vi "Scan_Dialog.vi"(0 "Acquisition Unit in (0)":i32, 1 "Acquire Definition":T9={"Acquire Mode"=enum."stop", "Acquisition mode"=enum."Sampled", "Acquirer"=enum."Cleverscope", "Transfer Chans"=enum."Chan A+B", "A max scale"=5.0, "A min scale"=-5.0, "B max scale"=5.0, "B min scale"=-5.0, "A Probe"=enum."x1", "B Probe"=enum."x1", "A Coupling"=enum."DC", "B Coupling"=enum."DC", "A Bandwidth"=1, "B Bandwidth"=1, "Trigger Source"=enum."Chan A", "Trigger Amplitude"=0.0, "A Trigger Amplitude"=0.0, "B Trigger Amplitude"=0.0, "Trigger Filter"=enum."None", "Trig Slope"=FALSE, "Trigger Holdoff"=0.0, "Dig Pattern Rqd"=FALSE, "Dig Pattern"=0, "Ext Trig Threshold"=0.0, "Dig Input Threshold"=0.0, "Start Time"=-0.003, "Stop Time"=0.003, "Pre Trig Time"=0.003, "Port"=enum."Port 1", "Num divisions"=6, "Num seq frames"=1, "Num Buffers"=2, "Sig Gen Freq"=1000.0, "Sig Gen Amp"=1.0, "Sig Gen Offset"=0.0, "Sig Gen Waveform"=enum."sine", "Sig Gen Sweep"=enum."Log", "Sig Gen Func"=enum."Standard", "Sig Gen Freq 2"=1000.0, "Sig Gen Phase"=180.0, "Trig 2 Function"=enum."None", "Min Trigger Period"=1e-08, "Max trigger Period"=0.0001, "Trigger count"=1, "Trig 2 Slope"=FALSE, "Trig 2 Source Chan"=enum."Chan A", "Trig 2 Level"=0.0, "Dig Pattern 2 Rqd"=FALSE, "Dig Pattern 2"=0, "Trigger 2 Source"=enum."Trigger 1 inverted", "Waveform Averages"=0, "Value changed"=0, "Freq Span"=0.0, "Freq Res"=0.0, "Duration"=0.0, "Resolution"=0.0, "Link Port"=enum."Debug", "Ext Sample Clock"=FALSE, "F Spare 2"=FALSE, "F Spare 3"=FALSE, "F Spare 4"=FALSE, "Sampler Resolution"=enum."10 bit", "Intf Source"=enum."USB", "Update Rate"=enum."20 Frame/sec", "Transfer Size"=enum."Normal", "Sig Gen Freq Step"=0.0, "TCP Adr"=0, "TCP port"=0, "CAU Ser Num Hi"=0, "CAU Ser Num Lo"=0, "Function Number"=0.0, "Function Parameter"=0.0, "Function Result"=0.0, "Link Start"=0, "Link Timebase"=0, "Link Timer"=0, "Link Setup"=0, "Spare 1"=0.0, "Spare 2"=0.0, "Spare 3"=0.0, "Spare 4"=0.0} {"Function Result" format="%#.6p"; "Function Parameter" format="%#.6p"; "Function Number" format="%#.6p"; "TCP Adr" format="%08x"; "Sig Gen Freq Step" format="%.2f"; "Sig Gen Phase" format="%.2f"; "Sig Gen Freq 2" format="%.2f"; "Resolution" format="%#.6p"; "Duration" format="%#.6p"; "Freq Res" format="%#.6p"; "Freq Span" format="%#.6p"; "Dig Pattern 2" format="%.0x"; "Trig 2 Level" step=0.001 format="%#.6p"; "Trigger count" step=1; "Max trigger Period" min=1e-08 max=42.9 step=0.01 format="%#.6p"; "Min Trigger Period" min=1e-08 max=42.9 step=0.01 format="%#_6p"; "Sig Gen Offset" format="%.2f"; "Sig Gen Amp" format="%.2f"; "Sig Gen Freq" format="%.2f"; "B Trigger Amplitude" format="%.1p"; "A Trigger Amplitude" format="%.1p"; "B Bandwidth" format="%x"; "A Bandwidth" format="%x"; "B min scale" format="%.2p"; "B max scale" format="%.2p"; "A min scale" format="%.2p"; "A max scale" format="%.2p"; "Trigger Holdoff" format="%.1p"; "Dig Input Threshold" format="%.2f"; "Ext Trig Threshold" format="%.2f"; "Dig Pattern" format="%.0x"; "Pre Trig Time" format="%.3p"; "Start Time" format="%.2p"; "Trigger Amplitude" format="%.1p"; "Stop Time" format="%.2p"}, 2 "Replay settings":T8={"Sampling Rate"=0.0, "Samples in replay"=0, "Replay Start Time"=1000.0, "Replay Stop Time"=0.003} {"Sampling Rate" format="%.3p"; "Samples in replay" format="%.3p"; "Replay Stop Time" format="%.3p"}, 5 "File Paths":T1, 9 "Scan Options":T5, 11 "error in":errorcluster, 12 "Scan Axis Config":T6, 13 "Index Axis Config":T6) -> (15 "error out":errorcluster)   [LabVIEW 2009]
uses:
  libraries/Cscope control driver.llb/Acquire Event type.ctl
  libraries/Cscope control driver.llb/Acquire capture type.ctl
  libraries/Cscope control driver.llb/Acquire capture method.ctl
  libraries/Cscope control driver.llb/Acquirer type.ctl
  libraries/Cscope control driver.llb/Input Range.ctl
  libraries/Cscope control driver.llb/Input Coupling.ctl
  libraries/Cscope control driver.llb/Input Bandwidth.ctl
  libraries/Cscope control driver.llb/USB channel.ctl
  libraries/Cscope control driver.llb/Trigger Filter.ctl
  libraries/Cscope control driver.llb/Cscope waveform type.ctl
  libraries/Cscope control driver.llb/Trigger Period.ctl
  libraries/Cscope control driver.llb/Trigger channel.ctl
  libraries/Cscope control driver.llb/Link port types.ctl
  libraries/Cscope control driver.llb/Acquirer resolution.ctl
  libraries/Cscope control driver.llb/Intf source.ctl
  libraries/Cscope control driver.llb/Acquire transfer size.ctl
  typedefs/Cscope/ReplaySettings.ctl
  typedefs/ScanAxisCfg.ctl
  typedefs/AxisSelect_Enum.ctl
  typedefs/SweepMode_Ring.ctl
  typedefs/ScanType.ctl
  typedefs/DwellTime.ctl
  typedefs/PathCluster.ctl
  typedefs/Ultra3000/IndexSettings_Cluster.ctl
  typedefs/Ultra3000/IndexType.ctl
  typedefs/Ultra3000/Index_Numeric.ctl
  typedefs/Ultra3000/HostControlModeRing.ctl
panel:
  in  "Channel Select":enum32{"Channel A", "Channel B", "Channel A+B"}(radio)
  out "Scan Line Progress":dbl(slide) scale=0.0..100.0 scale format="%#.0f"
  out "Total Progress":dbl(slide) scale=0.0..100.0 scale format="%#.0p"
  out "Num Points":i32
  out "dt":dbl
  out "Waveform Graph":waveform(sgl)[](graph)
  out "Status":string caption="Status \nMessage"
  in  "Stop":bool
  in  "Pause":bool
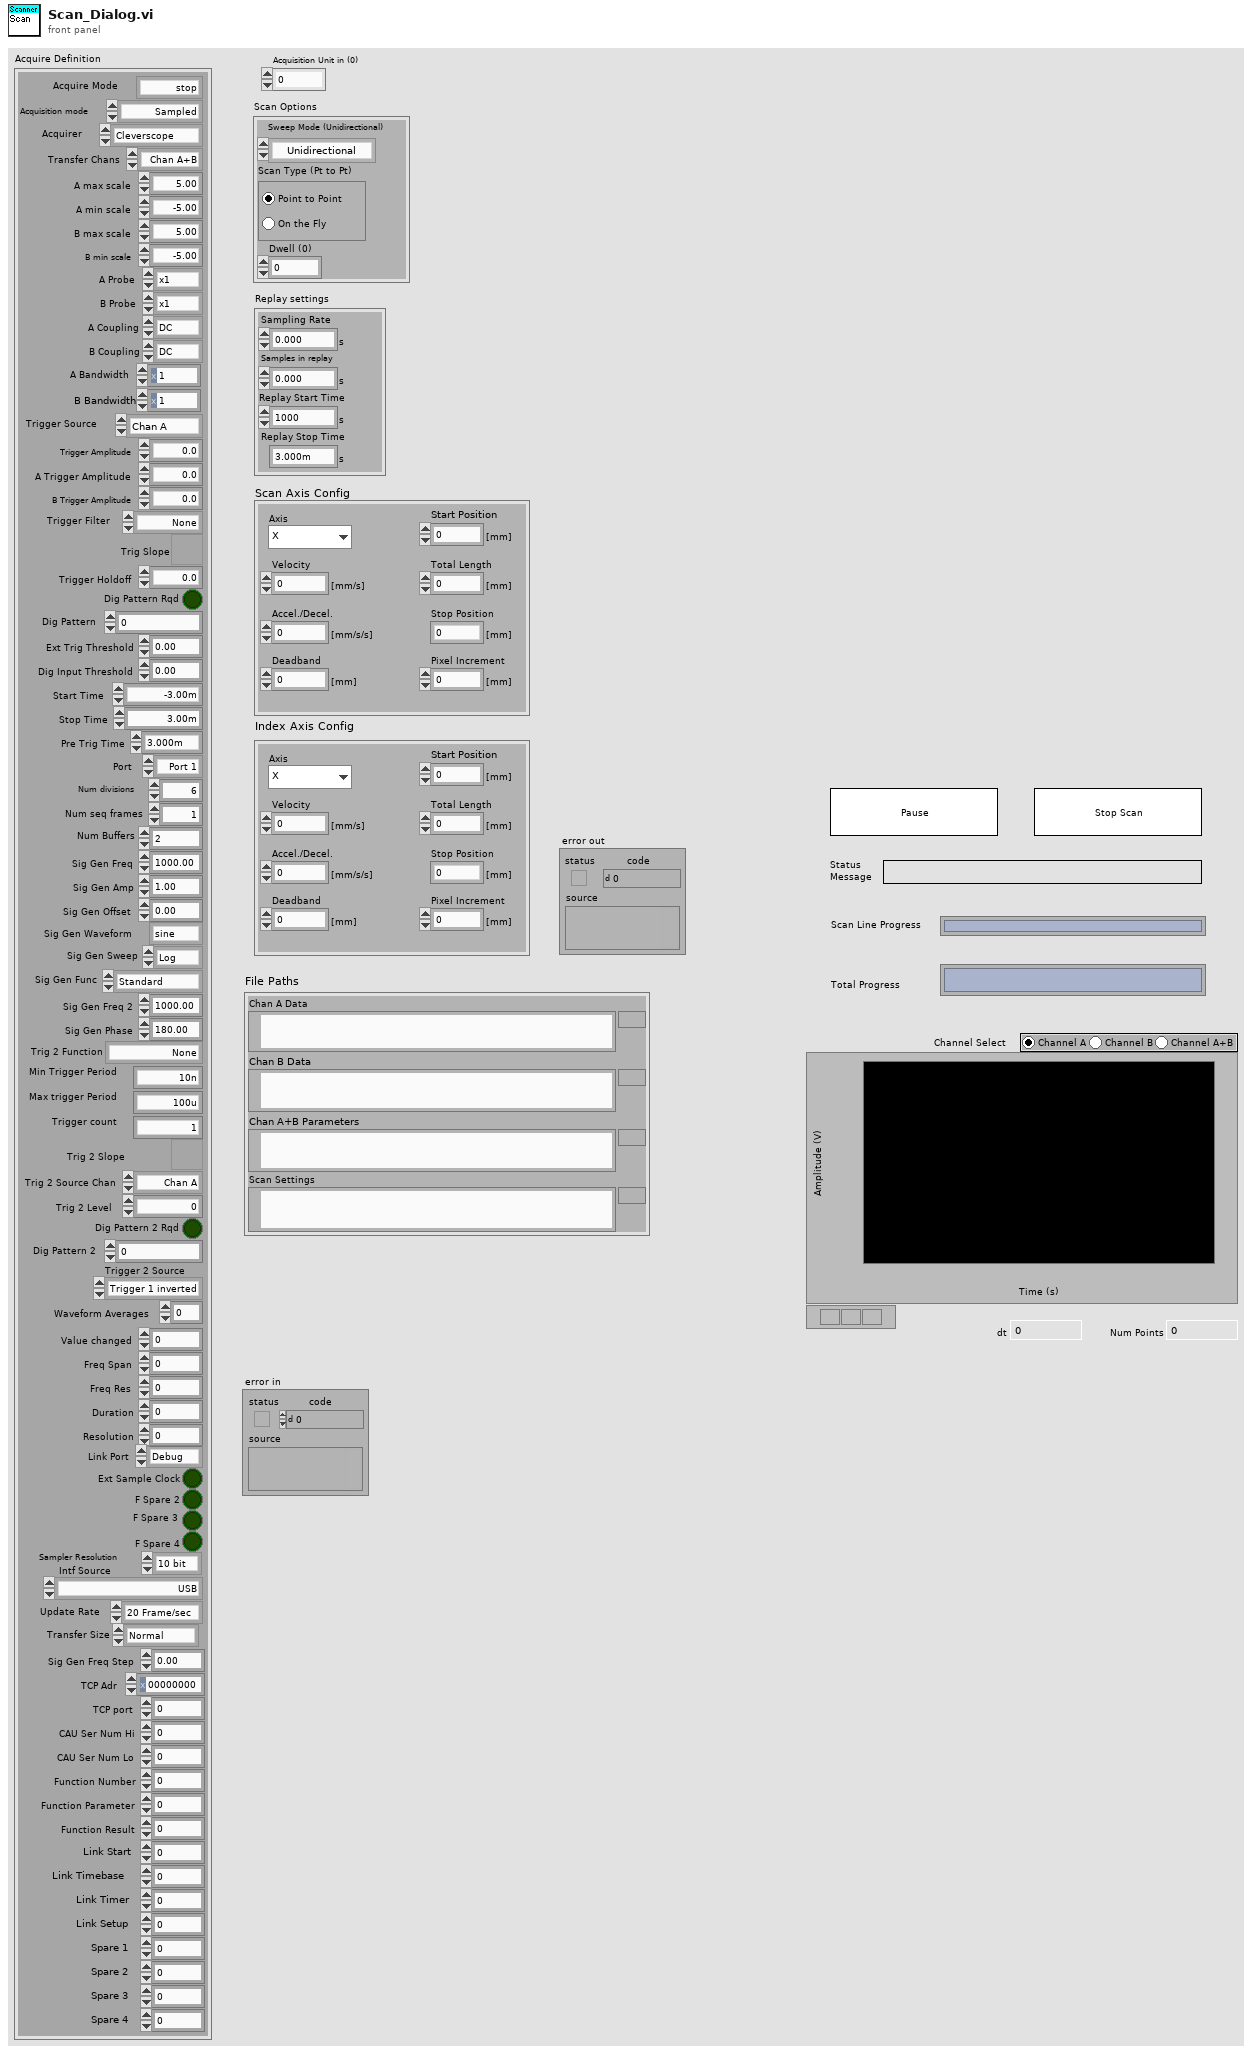
[diagram p1: front panel]
types:
  T1 = typedef "PathCluster.ctl" = cluster{"Chan A Data":path, "Chan B Data":path, "Chan A+B Parameters":path, "Scan Settings":path}
  T2 = typedef "SweepMode_Ring.ctl" = enum16{"Unidirectional", "Bidirectional"}
  T3 = typedef "ScanType.ctl" = enum32{"Point to Point", "On the Fly"}
  T4 = typedef "DwellTime.ctl" = u16
  T5 = cluster{"Sweep Mode (Unidirectional)":T2, "Scan Type (Pt to Pt)":T3, "Dwell (0)":T4}
  T6 = typedef "ScanAxisCfg.ctl" = cluster{"Axis ":T7, "Velocity":dbl, "Accel./Decel.":dbl, "Deadband":dbl, "Start Position":dbl, "Total Length":dbl, "Stop Position":dbl, "Pixel Increment":dbl}
  T7 = typedef "AxisSelect_Enum.ctl" = enum16{"X", "Y", "Z", "Axis Space"}
  T8 = typedef "ReplaySettings.ctl" = cluster{"Sampling Rate":dbl, "Samples in replay":u32, "Replay Start Time":dbl, "Replay Stop Time":dbl}
  T9 = typedef "Acquire Event type.ctl" = cluster{"Acquire Mode":T10, "Acquisition mode":T11, "Acquirer":T12, "Transfer Chans":enum16{"Chan A", "Chan B", "Chan A+B"}, "A max scale":dbl, "A min scale":dbl, "B max scale":dbl, "B min scale":dbl, "A Probe":T13, "B Probe":T13, "A Coupling":T14, "B Coupling":T14, "A Bandwidth":T15, "B Bandwidth":T15, "Trigger Source":T16, "Trigger Amplitude":dbl, "A Trigger Amplitude":dbl, "B Trigger Amplitude":dbl, "Trigger Filter":T17, "Trig Slope":bool, "Trigger Holdoff":dbl, "Dig Pattern Rqd":bool, "Dig Pattern":u32, "Ext Trig Threshold":dbl, "Dig Input Threshold":dbl, "Start Time":dbl, "Stop Time":dbl, "Pre Trig Time":dbl, "Port":enum16{"Port 1", "Port 2", "Port 3", "Port 4", "Port 5", "Port 6"}, "Num divisions":i16, "Num seq frames":i16, "Num Buffers":i32, "Sig Gen Freq":dbl, "Sig Gen Amp":dbl, "Sig Gen Offset":dbl, "Sig Gen Waveform":T18, "Sig Gen Sweep":enum16{"Linear", "Log"}, "Sig Gen Func":enum16{"Standard", "Auto advance", "Freq mod In8", "Phase mod In8"}, "Sig Gen Freq 2":dbl, "Sig Gen Phase":dbl, "Trig 2 Function":T19, "Min Trigger Period":dbl, "Max trigger Period":dbl, "Trigger count":u32, "Trig 2 Slope":bool, "Trig 2 Source Chan":T20, "Trig 2 Level":dbl, "Dig Pattern 2 Rqd":bool, "Dig Pattern 2":u32, "Trigger 2 Source":enum16{"Trigger 1 inverted", "Trig 2 Defn"}, "Waveform Averages":i32, "Value changed":i32, "Freq Span":dbl, "Freq Res":dbl, "Duration":dbl, "Resolution":dbl, "Link Port":T21, "Ext Sample Clock":bool, "F Spare 2":bool, "F Spare 3":bool, "F Spare 4":bool, "Sampler Resolution":T22, "Intf Source":T23, "Update Rate":enum16{"20 Frame/sec", "10 Frame/sec", "5 Frame/sec"}, "Transfer Size":T24, "Sig Gen Freq Step":dbl, "TCP Adr":u32, "TCP port":u32, "CAU Ser Num Hi":u32, "CAU Ser Num Lo":u32, "Function Number":dbl, "Function Parameter":dbl, "Function Result":dbl, "Link Start":u32, "Link Timebase":u32, "Link Timer":u32, "Link Setup":u32, "Spare 1":dbl, "Spare 2":dbl, "Spare 3":dbl, "Spare 4":dbl}
  T10 = typedef "Acquire capture type.ctl" = enum16{"single", "automatic", "triggered", "stop", "single stop", "replay"}
  T11 = typedef "Acquire capture method.ctl" = enum16{"Sampled", "Peak Captured", "Filtered", "Repetitive", "Waveform avg"}
  T12 = typedef "Acquirer type.ctl" = enum16{"Internal Sig Gen", "APC 901", "APC 901A", "Sound Card", "Cleverscope"}
  T13 = typedef "Input Range.ctl" = enum16{"x1", "x10", "x100", "x1K", "x20", "x50", "x200"}
  T14 = typedef "Input Coupling.ctl" = enum16{"AC", "DC"}
  T15 = typedef "Input Bandwidth.ctl" = u16
  T16 = typedef "USB channel.ctl" = enum32{"Chan A", "Chan B", "Ext Trigger", "Dig Trig", "Link Input", "chan_5", "chan_6", "chan_7", "chan_8", "chan_9", "chan_10", "chan_11", "chan_12", "chan_13", "chan_14", "chan_15"}
  T17 = typedef "Trigger Filter.ctl" = enum16{"None", "Low Pass", "Hi Pass", "Noise"}
  T18 = typedef "Cscope waveform type.ctl" = enum16{"sine", "triangle", "square", "DC", "OFF"}
  T19 = typedef "Trigger Period.ctl" = enum16{"None", "Trig 1~2 < min", "min<T1~2 < max", "Trig 1~2 > max", "Count Trig 1", "Count Trig 2"}
  T20 = typedef "Trigger channel.ctl" = enum32{"Chan A", "Chan B", "Ext Trigger", "Dig Trig", "Link Input"}
  T21 = typedef "Link port types.ctl" = enum8{"Debug", "Link Out", "Disabled", "Slave", "Master", "Uart", "SPI", "I2C", "Digital", "Sig Gen"}
  T22 = typedef "Acquirer resolution.ctl" = enum16{"10 bit", "12 Bit", "14 bit"}
  T23 = typedef "Intf source.ctl" = enum16{"USB", "Ethernet - Find by IP address", "Ethernet - Find first IP address", "Ethernet - Find by serial number"}
  T24 = typedef "Acquire transfer size.ctl" = enum16{"Normal", "100% Buffer", "50% Buffer", "10% Buffer", "5% Buffer", "2% Buffer", "Sequence"}
  T25 = typedef "Index_Numeric.ctl" = u8
  T26 = typedef "IndexSettings_Cluster.ctl" = cluster{"Type":T27, "Dwell":T4, "Velocity":dbl, "Accel/Decel":dbl}
  T27 = typedef "IndexType.ctl" = i32
  T28 = typedef "HostControlModeRing.ctl" = u16
  T29 = enum16{"big-endian, network order", "native, host order", "little-endian"}
  T30 = typedef "QSig_T0dt.ctl" = cluster{"T0":dbl, "dt":dbl, "n":i32}
  T31 = typedef "Cscope real.ctl" = sgl
  T32 = cluster{"Chan A Data":T31[], "Chan B Data":T31[]}
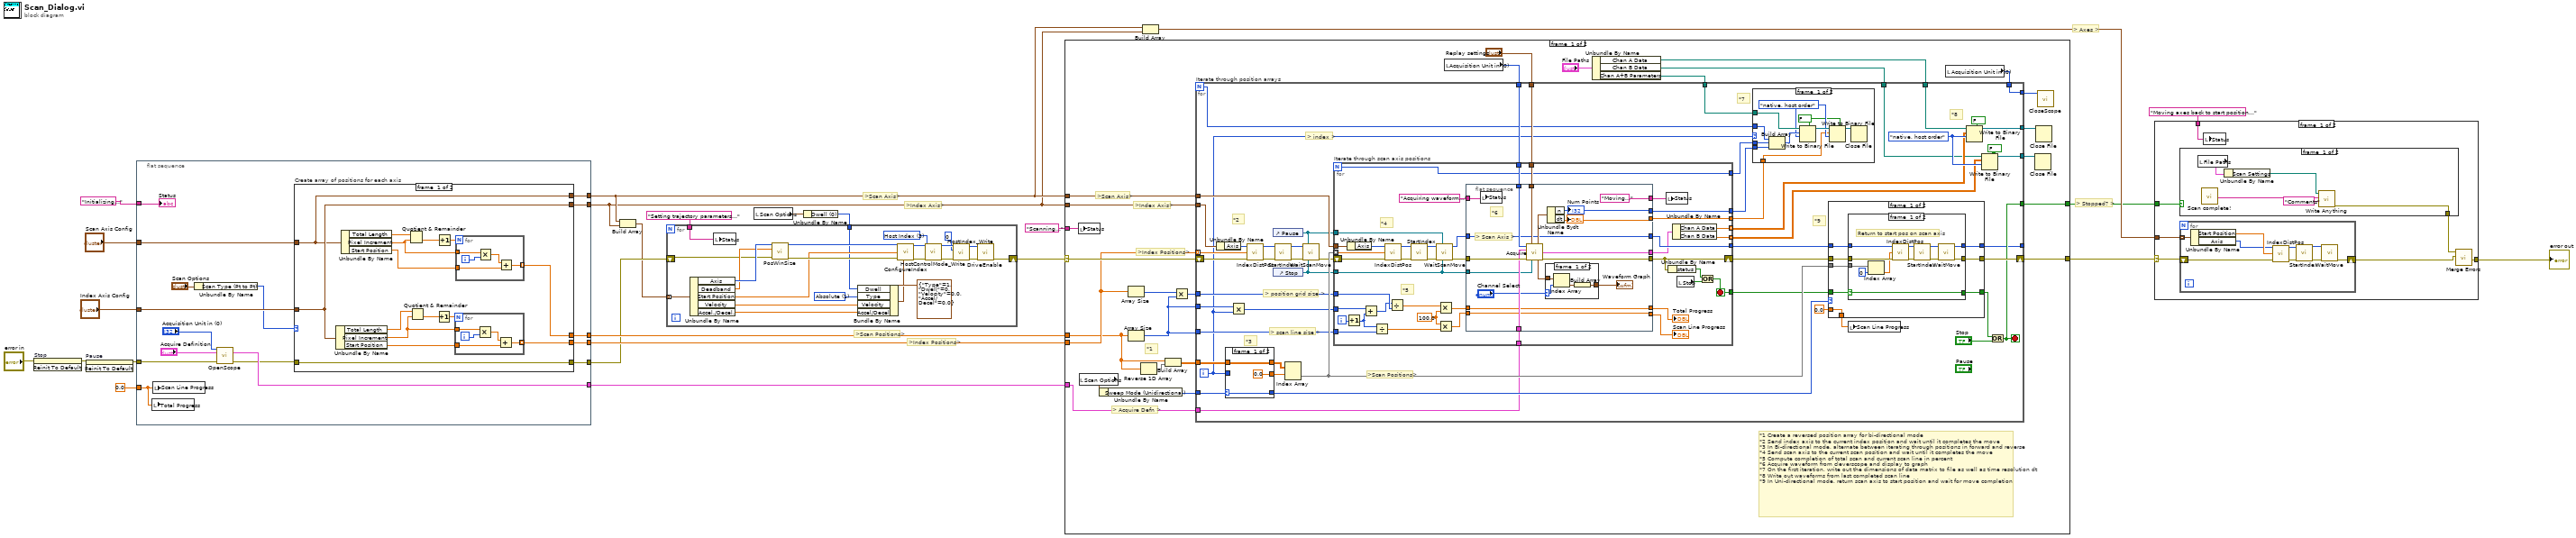
[diagram p0: block diagram]
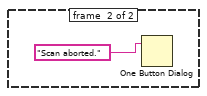
[diagram p2: hidden frame]
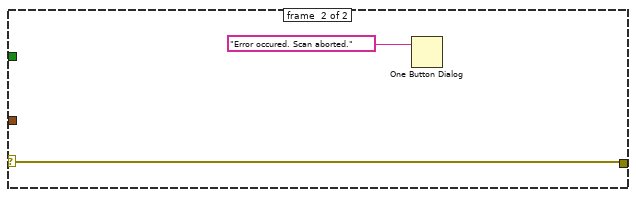
[diagram p3: hidden frame]
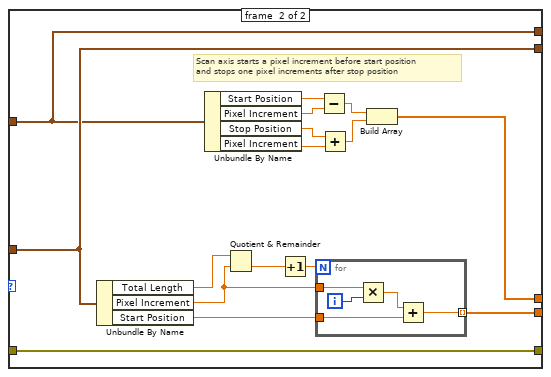
[diagram p4: hidden frame]
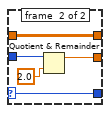
[diagram p6: hidden frame]
diagram:
  # "> Axes >"
  # "> Stopped? >"
  # ">Index Positions>"
  # ">Scan Positions>"
  # ">Index Axis>"
  # ">Scan Axis>"
  n1 = invoke on="Stop" class="Bool (strict)" method="Reinit To Default"(error in="error in") -> (error out=w5:errorcluster)  [unwired: 2 in, 2 out]
  n2 = invoke on="Pause" class="Bool (strict)" method="Reinit To Default"(error in=w5) -> (error out=w3:errorcluster)  [unwired: 2 in, 2 out]
  n3 = flat-sequence {
    tunnel: "Index Axis Config" -> [w40]
    tunnel: "Scan Axis Config" -> [w39]
    tunnel: [w38] -> w20
    tunnel: [w37] -> w19
    tunnel: [w36] -> w21
    tunnel: [w35] -> w22
    tunnel: [w32] -> w18
    tunnel: [w33] -> w6
    tunnel: "Initializing..." ("Status") -> [w31]
    tunnel: w3 -> [w29]
    tunnel: 0.0 ("Scan Line Progress") -> [w25]
    frame #0 {
      n4 = local write "Total Progress"(w25) -> ()
      n5 = local write "Scan Line Progress"(w25) -> ()
      n6 = Unbundle By Name("Scan Options") -> ("Scan Type (Pt to Pt)"=w26:T3)
      n7 = call "OpenScope.vi"("Acquisition Unit in (0)"="Acquisition Unit in (0)", "Acquire Defn In"="Acquire Definition", "error in"=w29) -> ("Acquire Defn Out"=w33:T9, "error out"=w28:errorcluster)  [unwired: 9 in, 2 out]
      n8 = case "Create array of positions for each axis" shown="\"Point to Point\", Default" w26 {
        tunnel: w40 -> [w45 w80]
        tunnel: w39 -> [w44 w79]
        tunnel: [w42 w81] -> w37
        tunnel: [w41 w66] -> w38
        tunnel: [w45 w80] -> w36
        tunnel: [w44 w79] -> w35
        tunnel: w28 -> [w43 w67]
        tunnel: [w43 w67] -> w32
        frame #0 {
          n9 = Unbundle By Name(w45) -> ("Total Length"=w49:dbl, "Pixel Increment"=w46:dbl, "Start Position"=w51:dbl)
          n10 = Unbundle By Name(w44) -> ("Total Length"=w53:dbl, "Pixel Increment"=w47:dbl, "Start Position"=w55:dbl)
          n11 = Quotient & Remainder(x=w53, y=w47) -> (floor(x/y)=w52:dbl)  [unwired: 1 out]
          n12 = Quotient & Remainder(x=w49, y=w46) -> (floor(x/y)=w48:dbl)  [unwired: 1 out]
          n13 = Increment(x=w48) -> (x+1=w50:dbl)
          n14 = Increment(x=w52) -> (x+1=w54:dbl)
          n15 = for {
            N: w50 -> [_]
            tunnel: w51 -> [w59]
            tunnel: w46 -> [w57]
            tunnel: [w56] -> w41 mode=indexing
            i -> [w60]
            n16 = Multiply(x=w57, y=w60) -> (x*y=w58:dbl)
            n17 = Add(x=w58, y=w59) -> (x+y=w56:dbl)
          }
          n18 = for {
            N: w54 -> [_]
            tunnel: w55 -> [w64]
            tunnel: w47 -> [w62]
            tunnel: [w61] -> w42 mode=indexing
            i -> [w65]
            n19 = Multiply(x=w62, y=w65) -> (x*y=w63:dbl)
            n20 = Add(x=w63, y=w64) -> (x+y=w61:dbl)
          }
        }
        frame #1 {
          # "Scan axis starts a pixel increment before start position \nand stops one pixel increments after stop position"
          n21 = Unbundle By Name(w80) -> ("Total Length"=w70:dbl, "Pixel Increment"=w69:dbl, "Start Position"=w68:dbl)
          n22 = Unbundle By Name(w79) -> ("Start Position"=w75:dbl, "Pixel Increment"=w74:dbl, "Stop Position"=w77:dbl, "Pixel Increment"=w78:dbl)
          n23 = Quotient & Remainder(x=w70, y=w69) -> (floor(x/y)=w71:dbl)  [unwired: 1 out]
          n24 = Increment(x=w71) -> (x+1=w72:dbl)
          n25 = for {
            N: w72 -> [_]
            tunnel: w68 -> [w85]
            tunnel: w69 -> [w83]
            tunnel: [w82] -> w66 mode=indexing
            i -> [w86]
            n26 = Multiply(x=w83, y=w86) -> (x*y=w84:dbl)
            n27 = Add(x=w84, y=w85) -> (x+y=w82:dbl)
          }
          n28 = Subtract(x=w75, y=w74) -> (x-y=w73:dbl)
          n29 = Add(x=w77, y=w78) -> (x+y=w76:dbl)
          n30 = Build Array(w73, w76) -> (w81:dbl[])
        }
      }
      "Status" <- w31
    }
  }
  n31 = Build Array(w22, w21) -> (w14:T6[])
  n32 = local read "Scan Options"() -> (w9:T5)
  n33 = Unbundle By Name(w9) -> ("Dwell (0)"=w8:T4)
  n34 = for {
    tunnel: w14 -> [w107] mode=indexing
    shift-right: [w91] -> w23
    shift-left: w18 -> [w90]
    tunnel: "Setting trajectory parameters..." ("Status") -> [w88]
    tunnel: w8 -> [w87]
    w92 = T28 3 items=["Normal Mode", "Setpoint velocity", "Setpoint current", "Host Index"] ("Host Control Mode (Normal)")
    w89 = T27 1 items=["Incremental", "Absolute", "Registration", "Jog"] ("Type")
    n35 = Unbundle By Name(w107) -> ("Axis"=w106:T7, "Deadband"=w104:dbl, "Start Position"=w100:dbl, "Velocity"=w101:dbl, "Accel./Decel."=w102:dbl)
    n36 = local write "Status"(w88) -> ()
    n37 = call "PosWinSize.vi"("Axis In"=w106, "Position Window Size"=w104, "error in (no error)"=w90) -> ("Axis Out"=w105:T7, "error out"=w103:errorcluster)  [unwired: 11 in]
    n38 = Bundle By Name(cluster=T26 {"Type"=1, "Dwell"=0, "Velocity"=0.0, "Accel/Decel"=0.0} ("Index Settings"), "Dwell"=w87, "Type"=w89, "Velocity"=w101, "Accel/Decel"=w102) -> (w108:T26)
    n39 = call "ConfigureIndex.vi"("Axis In"=w105, "Position"=w100, "error in (no error)"=w103, "Index Settings"=w108) -> ("Axis Out"=w98:T7, "error out"=w97:errorcluster)  [unwired: 9 in, 1 out]
    n40 = call "HostControlMode_Write.vi"("Axis In"=w98, "Host Control Mode (Normal)"=w92, "error in (no error)"=w97) -> ("Axis Out"=w99:T7, "error out"=w96:errorcluster)  [unwired: 11 in]
    n41 = call "HostIndex_Write.vi"("Axis In (Axis Space)"=w99, "Index"=T25 0, "error in (no error)"=w96) -> ("Axis Out"=w93:T7, "error out"=w94:errorcluster)  [unwired: 10 in, 1 out]
    n42 = call "DriveEnable.vi"("Axis In (Axis Space)"=w93, "error in (no error)"=w94) -> ("error out"=w91:errorcluster)  [unwired: 12 in, 1 out]
  }
  n43 = case shown="No Error" w23 {
    selector: w23 -> [w131 w296]
    tunnel: w20 -> [w124 _]
    tunnel: [w130 w296] -> w2
    tunnel: w19 -> [w123 _]
    tunnel: w21 -> [w133 _]
    tunnel: w22 -> [w132 _]
    tunnel: w6 -> [w129 _]
    tunnel: "Scanning..." ("Status") -> [w126 _]
    tunnel: [w125 _] -> w10
    frame #0 {
      # "*1"
      # "> Acquire Defn >"
      # ">Index Positions>"
      # ">Index Axis>"
      # ">Scan Axis>"
      # "*1 Create a reversed position array for bi-directional mode\n*2 Send index axis to the current index position and wait until it completes the move\n*3 In Bi-directional mode, alternate between iterating through positions in forward and reverse\n*4 Send scan axis to the current scan position and wait until it completes the move\n*5 Compute completion of total scan and current scan line in percent\n*6 Acquire waveform from cleverscope and display to graph\n*7 On the first iteration, write out the dimensions of data matrix to file as well as time resolution dt\n*8 Write out waveforms from last completed scan line\n*9 In Uni-directional mode, return scan axis to start position and wait for move completion"
      n44 = local write "Status"(w126) -> ()
      n45 = local read "Scan Options"() -> (w119:T5)
      n46 = Unbundle By Name(w119) -> ("Sweep Mode (Unidirectional)"=w118:T2)
      n47 = Array Size(array=w124) -> (size(s)=w116:i32)
      n48 = Array Size(array=w123) -> (size(s)=w115:i32)
      n49 = Reverse 1D Array(array=w123) -> (reversed array=w135:dbl[])
      n50 = Build Array(w123, w135) -> (w134:dbl[][])
      n51 = Multiply(x=w116, y=w115) -> (x*y=w122:i32)
      n52 = local read "Acquisition Unit in (0)"() -> (w127:i32)
      n53 = Unbundle By Name("File Paths") -> ("Chan A Data"=w114:path, "Chan B Data"=w113:path, "Chan A+B Parameters"=w112:path)
      n54 = local read "Acquisition Unit in (0)"() -> (w111:i32)
      n55 = for "Iterate through position arrays" {
        N -> [w147]
        tunnel: w124 -> [w186] mode=indexing
        tunnel: w133 -> [w184]
        tunnel: w132 -> [w183]
        tunnel: w134 -> [w178]
        tunnel: w118 -> [w177]
        shift-right: [w166] -> w130
        shift-left: w131 -> [w165]
        tunnel: w129 -> [w164]
        tunnel: "Replay settings" -> [w163]
        tunnel: w127 -> [w162]
        tunnel: [w159] -> w125
        tunnel: w122 -> [w158]
        tunnel: w115 -> [w157]
        tunnel: [w153] -> w121
        tunnel: [w152] -> w120
        tunnel: w112 -> [w138]
        tunnel: w115 -> [w145]
        tunnel: w114 -> [w140]
        tunnel: w113 -> [w139]
        tunnel: [w137] -> _
        tunnel: [w136] -> w110
        tunnel: w111 -> [w136]
        i -> [w144]
        stop <- w159 stop-if-true
        w156 = T29."native, host order" ("byte order (0:big-endian, network order)")
        # "> scan line size >"
        # "> position grid size >"
        # "> index >"
        # "*9"
        # "*8"
        # "*7"
        # "*3"
        # "*2"
        # ">Scan Positions>"
        n56 = Unbundle By Name(w184) -> ("Axis"=w185:T7)
        n57 = case shown="\"Bidirectional\"" w177 {
          selector: w177 -> [w197 w200]
          tunnel: w178 -> [w199 w201]
          tunnel: w144 -> [_ w203]
          tunnel: [0.0 w202] -> w176
          tunnel: [w199 w201] -> w175
          tunnel: [w197 w200] -> w173
          frame #0 {
          }
          frame #1 {
            n58 = Quotient & Remainder(x=w203, y=2.0) -> (x-y*floor(x/y)=w202:dbl)  [unwired: 1 out]
          }
        }
        n59 = Multiply(x=w145, y=w144) -> (x*y=w143:i32)
        n60 = call "IndexDistPos.vi"("Axis In"=w185, "Position"=w186, "error in (no error)"=w165) -> ("Axis Out"=w181:T7, "error out"=w182:errorcluster)  [unwired: 10 in, 1 out]
        n61 = control-ref of="Pause"() -> (w161:refnum<vi>)
        n62 = control-ref of="Stop"() -> (w160:refnum<vi>)
        n63 = call "StartIndex.vi"("Axis In (Axis Space)"=w181, "error in (no error)"=w182) -> ("Axis Out"=w172:T7, "error out"=w171:errorcluster)  [unwired: 12 in]
        n64 = Index Array(array=w175, index (row)=w176) -> (element=w174:dbl[])  [unwired: 1 in]
        n65 = call "WaitScanMove.vi"("Axis In"=w172, "Pause"=w161, "error in (no error)"=w171, "Stop"=w160) -> ("error out"=w170:errorcluster)  [unwired: 10 in, 1 out]
        n66 = for "Iterate through scan axis positions" {
          N -> [w239]
          tunnel: w174 -> [w269] mode=indexing
          shift-right: [w264] -> w180
          shift-left: w170 -> [w270]
          tunnel: w183 -> [w272]
          tunnel: [w245] -> w179
          tunnel: [w268] -> w169
          tunnel: w164 -> [w263]
          tunnel: w163 -> [w262]
          tunnel: w162 -> [w261]
          tunnel: w161 -> [w259]
          tunnel: w160 -> [w258]
          tunnel: w143 -> [w255]
          tunnel: w158 -> [w254]
          tunnel: w157 -> [w250]
          tunnel: [w242] -> w155 mode=indexing
          tunnel: [w241] -> w154 mode=indexing
          tunnel: [w240] -> w149
          tunnel: [w239] -> w148
          tunnel: [w238] -> w146
          i -> [w233]
          stop <- w268 stop-if-true
          w252 = 100.0 ("y")
          # "*5"
          # "*4"
          n67 = Increment(x=w233) -> (x+1=w232:i32)
          n68 = Unbundle By Name(w272) -> ("Axis"=w271:T7)
          n69 = Add(x=w255, y=w232) -> (x+y=w253:i32)
          n70 = Divide(x=w232, y=w250) -> (x/y=w251:dbl)
          n71 = call "IndexDistPos.vi"("Axis In"=w271, "Position"=w269, "error in (no error)"=w270) -> ("Axis Out"=w249:T7, "error out"=w248:errorcluster)  [unwired: 10 in, 1 out]
          n72 = Divide(x=w253, y=w254) -> (x/y=w256:dbl)
          n73 = call "StartIndex.vi"("Axis In (Axis Space)"=w249, "error in (no error)"=w248) -> ("Axis Out"=w247:T7, "error out"=w246:errorcluster)  [unwired: 12 in]
          n74 = call "WaitScanMove.vi"("Axis In"=w247, "Pause"=w259, "error in (no error)"=w246, "Stop"=w258) -> ("Axis Out"=w244:T7, "error out"=w266:errorcluster)  [unwired: 10 in]
          n75 = Multiply(x=w256, y=w252) -> (x*y=w237:dbl)
          n76 = Multiply(x=w252, y=w251) -> (x*y=w235:dbl)
          n77 = flat-sequence {
            tunnel: w266 -> [w290]
            tunnel: [w289] -> w264
            tunnel: w263 -> [w288]
            tunnel: w262 -> [w287]
            tunnel: w261 -> [w286]
            tunnel: ["Moving..." ("Status")] -> w260
            tunnel: w258 -> [w284]
            tunnel: "Acquiring waveform..." ("Status") -> [w283]
            tunnel: [w281] -> w245
            tunnel: w244 -> [w281]
            tunnel: [w280] -> w243
            tunnel: [w277] -> w240
            tunnel: [w276] -> w238
            tunnel: [w279] -> w236
            tunnel: w237 -> [w279]
            tunnel: [w278] -> w234
            tunnel: w235 -> [w278]
            frame #0 {
              # "*6"
              # "> Scan Axis >"
              n78 = local write "Status"(w283) -> ()
              n79 = call "Acquire.vi"("Acquisition Unit in (0)"=w286, "Replay settings"=w287, "Acquire Definition"=w288, "error in (no error)"=w290, "Stop Refnum"=w284) -> ("T0dt"=w282:T30, "Chan AB Data"=w280:T32, "Waveform"=w275:waveform(sgl)[], "error out"=w289:errorcluster)  [unwired: 5 in, 2 out]
              n80 = case shown="\"Channel A+B\"" "Channel Select" {
                selector: "Channel Select" -> [w293 _]
                tunnel: w275 -> [w294 w295]
                tunnel: [w291 w295] -> w274
                frame #0 {
                  n81 = Index Array(array=w294, index=w293) -> (element=w292:waveform(sgl))
                  n82 = Build Array(w292) -> (w291:waveform(sgl)[])
                }
                frame #1 {
                }
              }
              "Waveform Graph" <- w274
              n83 = Unbundle By Name(w282) -> ("n"=w276:i32, "dt"=w277:dbl)
              "dt" <- w277
              "Num Points" <- w276
            }
          }
          n84 = local write "Status"(w260) -> ()
          n85 = Unbundle By Name(w264) -> ("status"=w265:bool)
          n86 = Unbundle By Name(w243) -> ("Chan A Data"=w242:T31[], "Chan B Data"=w241:T31[])
          n87 = local read "Stop"() -> (w267:bool)
          n88 = Or(x=w265, y=w267) -> (x .or. y?=w268:bool)
          "Total Progress" <- w236
          "Scan Line Progress" <- w234
        }
        n89 = case shown="0" w144 {
          tunnel: w138 -> [w196 _]
          tunnel: w149 -> [w188 _]
          tunnel: w148 -> [w194 _]
          tunnel: w147 -> [w195 _]
          tunnel: w146 -> [w189 _]
          frame #0 {
            w191 = T29."native, host order" ("byte order (0:big-endian, network order)")
            w190 = FALSE ("prepend array or string size? (T)")
            n90 = Build Array(w195, w194, w189) -> (w193:i32[])
            n91 = Write to Binary File(file (use dialog)=w196, data=w193, 5:w190, 9:w191) -> (refnum out=w192:refnum<file>)  [unwired: 2 in, 2 out]
            n92 = Write to Binary File(file (use dialog)=w192, data=w188, 5:w190, 9:w191) -> (refnum out=w187:refnum<file>)  [unwired: 2 in, 2 out]
            n93 = Close File(refnum=w187) -> ()  [unwired: 1 in, 2 out]
          }
          frame #1 {
          }
        }
        n94 = case shown="\"Unidirectional\", Default" w173 {
          tunnel: [w211 w231] -> w166
          tunnel: w180 -> [w212 w231]
          tunnel: w169 -> [w208 w230]
          tunnel: w179 -> [w210 w228]
          tunnel: w174 -> [w209 _]
          tunnel: [w207 w230] -> w168
          tunnel: [w206 w229] -> w141
          tunnel: 0.0 ("Scan Line Progress") -> [w206 w229]
          tunnel: [w205 w228] -> w137
          frame #0 {
            n95 = case shown="False" w208 {
              selector: w208 -> [w218 w227]
              tunnel: w212 -> [w224 w226]
              tunnel: [w215 w226] -> w211
              tunnel: w210 -> [w221 w225]
              tunnel: w209 -> [w217 _]
              tunnel: [w218 w227] -> w207
              tunnel: [w213 w225] -> w205
              frame #0 {
                # "Return to start pos on scan axis"
                n96 = Index Array(array=w217, index=0) -> (element=w219:dbl)
                n97 = call "IndexDistPos.vi"("Axis In"=w221, "Position"=w219, "error in (no error)"=w224) -> ("Axis Out"=w222:T7, "error out"=w223:errorcluster)  [unwired: 10 in, 1 out]
                n98 = call "StartIndex.vi"("Axis In (Axis Space)"=w222, "error in (no error)"=w223) -> ("Axis Out"=w214:T7, "error out"=w216:errorcluster)  [unwired: 12 in]
                n99 = call "WaitMove.vi"("Axis In"=w214, "error in (no error)"=w216) -> ("Axis Out"=w213:T7, "error out"=w215:errorcluster)  [unwired: 12 in]
              }
              frame #1 {
              }
            }
          }
          frame #1 {
          }
        }
        n100 = local write "Scan Line Progress"(w141) -> ()
        n101 = Write to Binary File(file (use dialog)=w140, data=w155, 5:FALSE ("prepend array or string size? (T)"), 9:w156) -> (refnum out=w153:refnum<file>)  [unwired: 2 in, 2 out]
        n102 = Write to Binary File(file (use dialog)=w139, data=w154, 5:FALSE ("prepend array or string size? (T)"), 9:w156) -> (refnum out=w152:refnum<file>)  [unwired: 2 in, 2 out]
        n103 = Or(x=w168, y="Stop") -> (x .or. y?=w159:bool)
      }
      n104 = Close File(refnum=w120) -> ()  [unwired: 1 in, 2 out]
      n105 = Close File(refnum=w121) -> ()  [unwired: 1 in, 2 out]
      n106 = call "CloseScope.vi"("Acquisition Unit in (0)"=w110) -> ()  [unwired: 8 in, 3 out]
    }
    frame #1 {
    }
  }
  n107 = Build Array(w22, w21) -> (w24:T6[])
  n108 = case shown="No Error" w2 {
    selector: w2 -> [w302 w320]
    tunnel: w24 -> [w303 _]
    tunnel: [w297 w320] -> w1
    tunnel: "Moving axes back to start position..." ("Status") -> [w301 _]
    tunnel: w10 -> [w300 _]
    frame #0 {
      n109 = case shown="False" w300 {
        tunnel: [w304 _] -> w299
        frame #0 {
          n110 = local read "File Paths"() -> (w308:T1)
          n111 = call "Scan complete!"() -> ("Comments:"=w306:string)  [unwired: 17 in, 2 out]
          n112 = Unbundle By Name(w308) -> ("Scan Settings"=w307:path)
          n113 = call "Write Anything.vi"("Section Name (Name of \"Anything\")"="Comments" ("Section Name (Name of \"Anything\")"), "Anything"=w306, "Path (dialog)"=w307) -> ("Error Out"=w304:errorcluster)  [unwired: 8 in]
        }
        frame #1 {
          n114 = One Button Dialog(message="Scan aborted.") -> ()  [unwired: 1 in, 1 out]
        }
      }
      n115 = for {
        shift-right: [w314] -> w298
        shift-left: w302 -> [w310]
        tunnel: w303 -> [w318] mode=indexing
        n116 = Unbundle By Name(w318) -> ("Start Position"=w312:dbl, "Axis"=w311:T7)
        n117 = call "IndexDistPos.vi"("Axis In"=w311, "Position"=w312, "error in (no error)"=w310) -> ("Axis Out"=w317:T7, "error out"=w316:errorcluster)  [unwired: 10 in, 1 out]
        n118 = call "StartIndex.vi"("Axis In (Axis Space)"=w317, "error in (no error)"=w316) -> ("Axis Out"=w313:T7, "error out"=w315:errorcluster)  [unwired: 12 in]
        n119 = call "WaitMove.vi"("Axis In"=w313, "error in (no error)"=w315) -> ("error out"=w314:errorcluster)  [unwired: 12 in, 1 out]
      }
      n120 = local write "Status"(w301) -> ()
      n121 = call <vilib>:"Merge Errors.vi"("error in 2 (no error)"=w298, "error in 1 (no error)"=w299) -> ("error out"=w297:errorcluster)  [unwired: 5 in]
    }
    frame #1 {
      n122 = One Button Dialog(message="Error occured. Scan aborted.") -> ()  [unwired: 1 in, 1 out]
    }
  }
  "error out" <- w1
